vi "Example 02c - Anonymous Functions.vi"() -> ()   [LabVIEW 2020]
uses:
  Lua for LabVIEW/Lua/Lua.lvclass
panel:
  out "scaled array":dbl[](array[numeric])
  in  "array":dbl[](array[numeric])=[3.0, -2.0, 1.0, 2.0]
  in  "scale":dbl=2.2
  out "error out":errorcluster
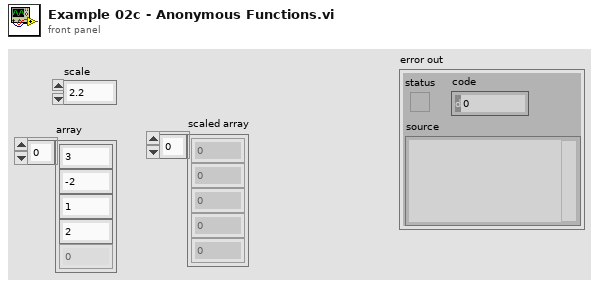
[diagram p1: front panel]
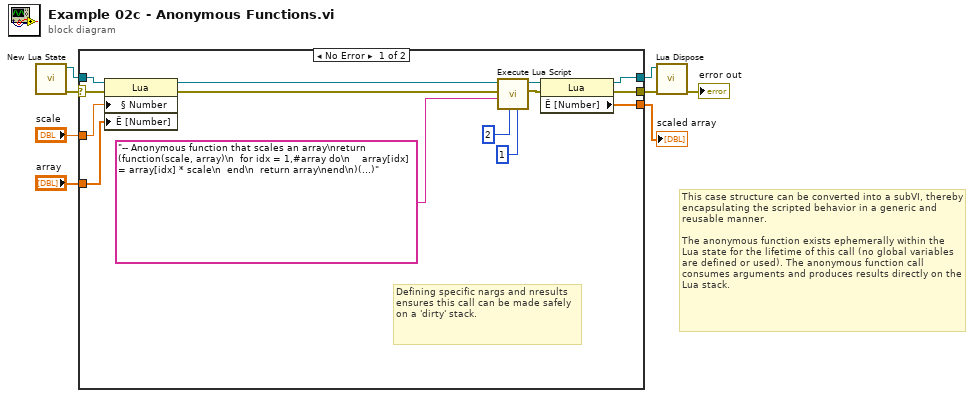
[diagram p0: block diagram]
diagram:
  # "This case structure can be converted into a subVI, thereby encapsulating the scripted behavior in a generic and reusable manner.\n\nThe anonymous function exists ephemerally within the Lua state for the lifetime of this call (no global variables are defined or used). The anonymous function call consumes arguments and produces results directly on the Lua stack."
  n1 = call "New Lua State.vi"() -> ("error out"=w7:errorcluster, "Lua out"=w8:refnum<class "Lua.lvclass">)  [unwired: 10 in]
  n2 = case shown="No Error" w7 {
    selector: w7 -> [w14 w23]
    tunnel: [w22 w23] -> w5
    tunnel: [w21 w24] -> w4
    tunnel: w8 -> [w20 w24]
    tunnel: "scale" -> [w19 _]
    tunnel: "array" -> [w18 _]
    tunnel: [w17 _] -> w1
    frame No Error {
      # "Defining specific nargs and nresults ensures this call can be made safely on a 'dirty' stack."
      n3 = property class="Lua"(reference=w20, error in=w14, "§ Number"=w19, "Ё [Number]"=w18) -> (reference out=w15:refnum<class "Lua.lvclass">, error out=w11:errorcluster)
      n4 = call-dynamic "Execute Lua Script.vi"("nresults"=1, "nargs"=2, "lua script"="-- Anonymous function that scales an array\nreturn (function(scale, array)\n  for idx = 1,#array do\n    array[idx] = array[idx] * scale\n  end\n  return array\nend\n)(...)", "error in (no error)"=w11, "Lua in"=w15) -> ("error out"=w10:errorcluster, "Lua out"=w16:refnum<class "Lua.lvclass">)  [unwired: 5 in]
      n5 = property class="Lua"(reference=w16, error in=w10) -> (reference out=w21:refnum<class "Lua.lvclass">, error out=w22:errorcluster, "Ё [Number]"=w17:dbl[])
    }
    frame Error {
    }
  }
  "scaled array" <- w1
  n6 = call-dynamic "Lua Dispose.vi"("error in (no error)"=w5, "Lua in"=w4) -> ("error out"=→"error out":errorcluster)  [unwired: 9 in]
